vi "Determine Clicked Array Element Index - Get Minimal Array Properties.vi"(0 "Array Reference":refnum<vi>, 4 "Coords of Click":T1, 5 "error in (no error)":errorcluster) -> (14 "dup Array Reference":refnum<vi>, 16 "Minimal Array Properties.Bounds":T3, 17 "Minimal Array Properties.Position":T2, 18 "dup Coords of Click":T1, 19 "error out":errorcluster)   [LabVIEW 2019]
doc: "Determine Clicked Array Element Index - Get Minimal Array Properties.vi\n\nDescription:\nThis VI returns the minimal properties of the array specified by the Array Reference input. Minimal properties are the properties when the scrollbars, index display, label and caption are hidden.\n\nInputs:\nArray Reference - Reference to the array to operate on.\n\nCoords of Click - The coordinates indicating where the user clicked.\n\nerror in - Standard error cluster.\n\nOutputs:\ndup Array Reference - Dup reference to the array to operate on.\n\nMinimal Array Properties.Bounds - The bounds of the array when the scrollbars, index display, label and caption are hidden.\n\nMinimal Array Properties.Position - The position of the array when the scrollbars, index display, label and caption are hidden.\n\ndup Coords of Click - Dup coordinates indicating where the user clicked.\n\nerror out - Standard error cluster.\n\nDeveloped By:\nMark.ridgley\nMark.Ridgley_LabVIEW.Developer@comcast.net"
uses:
  <vilib>/Utility/miscctls.llb/LVBoundsTypeDef.ctl
  <vilib>/Utility/miscctls.llb/LVPositionTypeDef.ctl
  <vilib>/Utility/miscctls.llb/LVPoint32TypeDef.ctl
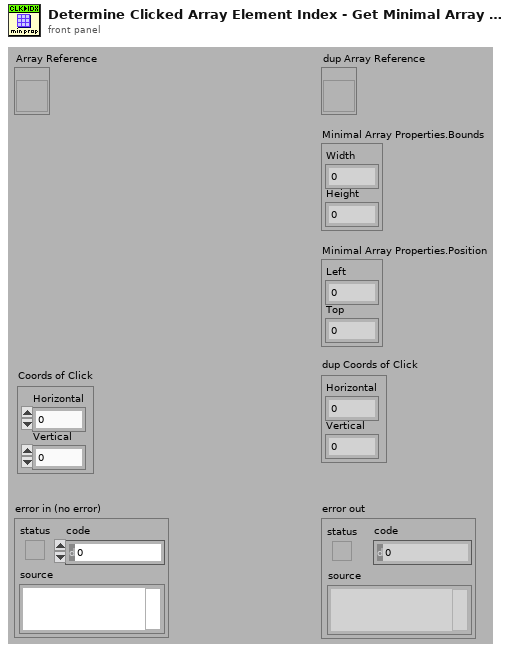
[diagram p1: front panel]
types:
  T1 = typedef "LVPoint32TypeDef.ctl" = cluster{"Horizontal":i32, "Vertical":i32}
  T2 = typedef "LVPositionTypeDef.ctl" = cluster{"Left":i32, "Top":i32}
  T3 = typedef "LVBoundsTypeDef.ctl" = cluster{"Width":u32, "Height":u32}
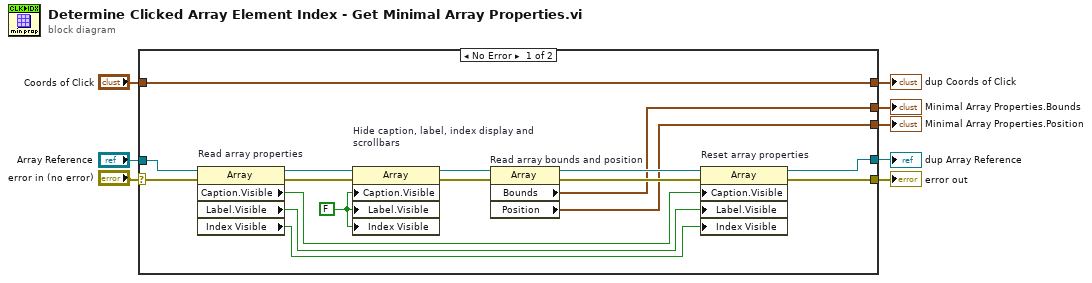
[diagram p0: block diagram]
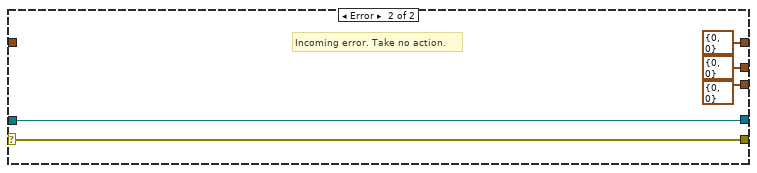
[diagram p2: hidden frame]
diagram:
  n1 = case shown="No Error" "error in (no error)" {
    selector: "error in (no error)" -> [w16 w30]
    tunnel: [w24 w29] -> w8
    tunnel: [w12 T3 {"Width"=0, "Height"=0}] -> w7
    tunnel: "Array Reference" -> [w21 w29]
    tunnel: [w17 T2 {"Left"=0, "Top"=0} ("Position")] -> w5
    tunnel: [w11 w30] -> w3
    tunnel: [w15 T1 {"Horizontal"=0, "Vertical"=0} ("Coords of Click")] -> w2
    tunnel: "Coords of Click" -> [w15 _]
    frame No Error {
      w13 = FALSE ("Label.Visible")
      n2 = property on="Read array properties" class="Array"(reference=w21, error in=w16) -> (reference out=w14:refnum<vi>, error out=w9:errorcluster, "Caption.Visible"=w18:bool, "Label.Visible"=w19:bool, "Index Visible"=w23:bool)
      n3 = property on="Hide caption, label, index display and scrollbars" class="Array"(reference=w14, error in=w9, "Caption.Visible"=w13, "Label.Visible"=w13, "Index Visible"=w13) -> (reference out=w22:refnum<vi>, error out=w10:errorcluster)
      n4 = property on="Read array bounds and position" class="Array"(reference=w22, error in=w10) -> (reference out=w20:refnum<vi>, error out=w25:errorcluster, "Bounds"=w12:T3, "Position"=w17:T2)
      n5 = property on="Reset array properties" class="Array"(reference=w20, error in=w25, "Caption.Visible"=w18, "Label.Visible"=w19, "Index Visible"=w23) -> (reference out=w24:refnum<vi>, error out=w11:errorcluster)
    }
    frame Error {
      # "Incoming error. Take no action."
    }
  }
  "dup Array Reference" <- w8
  "Minimal Array Properties.Bounds" <- w7
  "Minimal Array Properties.Position" <- w5
  "error out" <- w3
  "dup Coords of Click" <- w2
